vi "Read Cooler ON_OFF.vi"(8 "error in (no error)":errorcluster, 11 "Cooler in":refnum<class "Cooler.lvclass">) -> (0 "error out":errorcluster, 2 "Cooler ON/OFF":u8, 3 "Cooler out":refnum<class "Cooler.lvclass">)   [LabVIEW 2018]
uses:
  Cooler.lvclass
  C:/Users/observer/Desktop/SPARC4_ACS/Simulated_Cooler/Simulated_Cooler.lvclass
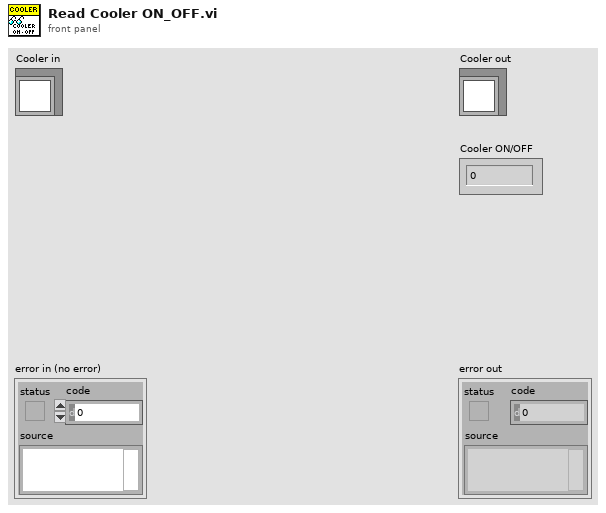
[diagram p1: front panel]
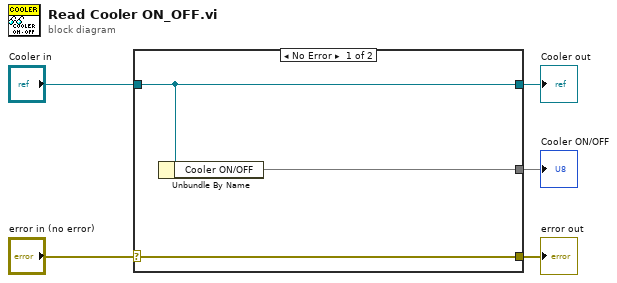
[diagram p0: block diagram]
diagram:
  n1 = case shown="No Error" "error in (no error)" {
    selector: "error in (no error)" -> [w8 w9]
    tunnel: [w8 w9] -> w4
    tunnel: [w7 w10] -> w2
    tunnel: "Cooler in" -> [w7 w10]
    tunnel: [w6 _] -> w1
    frame No Error {
      n2 = Unbundle By Name(w7) -> ("Cooler ON/OFF"=w6)
    }
    frame Error {
    }
  }
  "error out" <- w4
  "Cooler out" <- w2
  "Cooler ON/OFF" <- w1
